vi "UpdateMatlabParamDataToVartiant.vi"(6 "Ignore parent name":bool, 8 "MatlabDataBundle":T1, 9 "curNameIndex":i32, 10 "NamePath":string[](array[string]), 11 "Type (or value to update)":variant) -> (3 "Value":variant)   [LabVIEW 2017]
uses:
  Types/MatlabDataBundle.ctl
  Types/MatlabDataType.ctl
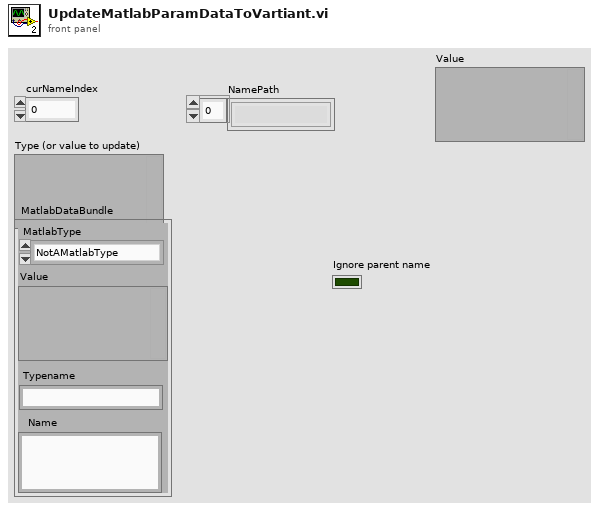
[diagram p1: front panel]
types:
  T1 = typedef "MatlabDataBundle.ctl" = cluster{"MatlabType":T2, "Value":variant, "Name":string, "Typename":string}
  T2 = typedef "MatlabDataType.ctl" = enum16{"NotAMatlabType", "Real", "Complex", "String", "Boolean"}
  T3 = typedef "NI_Data Type.lvlib/Data Type.ctl" = enum8{"Invalid Type", "Void", "I8", "I16", "I32", "I64", "U8", "U16", "U32", "U64", "Single Float", "Double Float", "Extended Float", "Single Complex", "Double Complex", "Extended Complex", "Enum U8", "Enum U16", "Enum U32", "Enum U64", "Single Float With Unit", "Double Float With Unit", "Extended Float With Unit", "Single Complex with Unit", "Double Complex with Unit", "Extended Complex with Unit", "Boolean", "String", "Path", "Picture", "Tag", "Array", "Cluster", "Variant", "LV Variant", "Waveform", "Timestamp", "Digital Waveform", "Digital Data", "ExpressData", "Refnum", "External Data", "VI", "Poly VI", "LabVIEW Class Instance", "Fixed Point"}
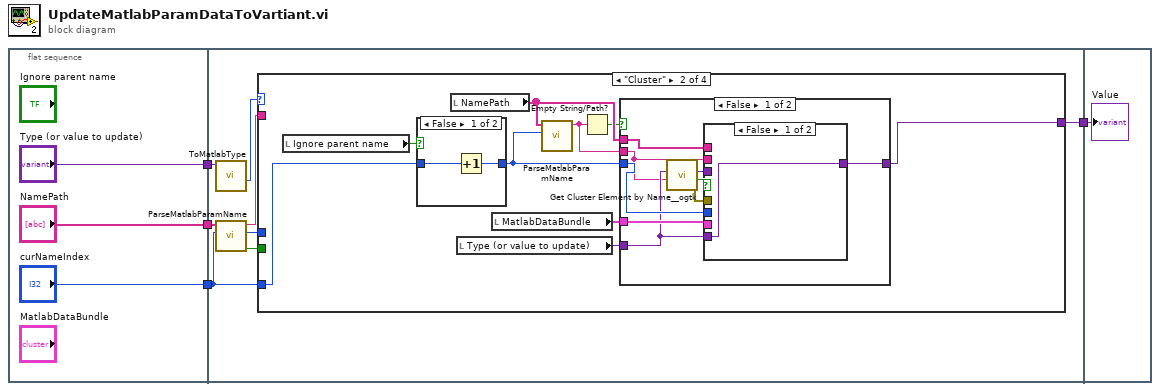
[diagram p0: block diagram]
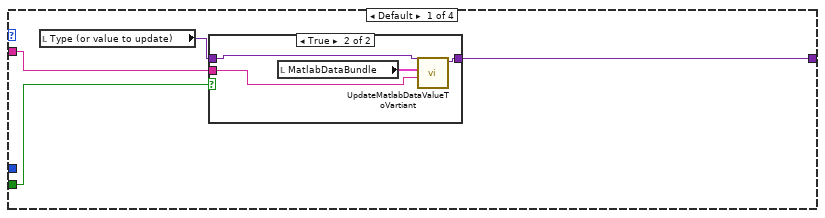
[diagram p2: hidden frame]
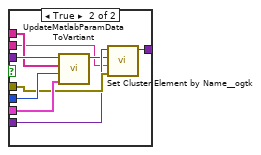
[diagram p4: hidden frame]
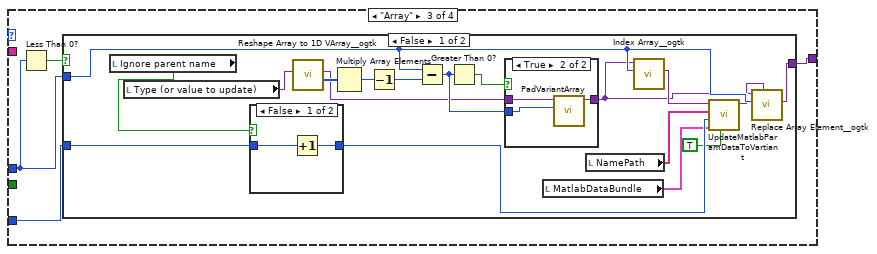
[diagram p7: hidden frame]
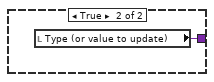
[diagram p10: hidden frame]
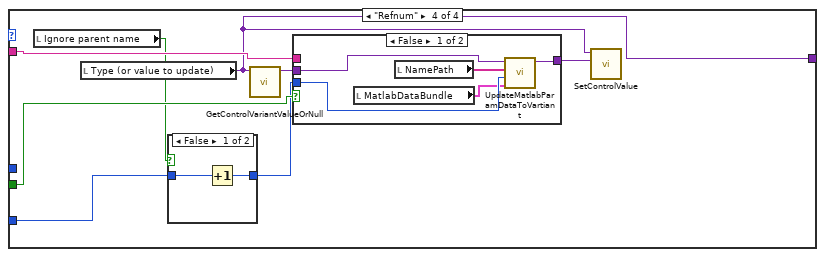
[diagram p11: hidden frame]
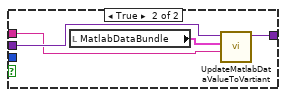
[diagram p13: hidden frame]
diagram:
  n1 = flat-sequence {
    tunnel: ["curNameIndex"] -> w4
    tunnel: ["Type (or value to update)"] -> w3
    tunnel: ["NamePath"] -> w2
    tunnel: w4 -> [w11]
    tunnel: w3 -> [w9]
    tunnel: w2 -> [w10]
    tunnel: [w8] -> w1
    tunnel: w1 -> [w107]
    frame #0 {
    }
    frame #1 {
      n2 = call "ToMatlabType.vi"("Value"=w9) -> ("Type"=w14:T3)  [unwired: 7 in, 3 out]
      n3 = call "ParseMatlabParamName.vi"("curNameIndex"=w11, "NamePath"=w10) -> ("At last name"=w15:bool, "Array Index (or -1)"=w12:i32, "Name"=w13:string)  [unwired: 6 in, 1 out]
      n4 = case shown="\"Cluster\"" w14 {
        tunnel: w15 -> [w18 _ _ w93]
        tunnel: [w19 w27 w59 w87] -> w8
        tunnel: w12 -> [_ _ w58 _]
        tunnel: w13 -> [w17 _ _ w89]
        tunnel: w11 -> [_ w33 w57 w94]
        frame Default {
          n5 = local read "Type (or value to update)"() -> (w16:variant)
          n6 = case shown="True" w18 {
            tunnel: [w20 w24] -> w19
            tunnel: w16 -> [w20 w23]
            tunnel: w17 -> [_ w22]
            frame False {
            }
            frame True {
              n7 = local read "MatlabDataBundle"() -> (w21:T1)
              n8 = call "UpdateMatlabDataValueToVartiant.vi"("name"=w22, "MatlabDataBundle"=w21, "Type (or value to update)"=w23) -> ("Value"=w24:variant)  [unwired: 8 in]
            }
          }
        }
        frame "Cluster" {
          n9 = local read "Ignore parent name"() -> (w30:bool)
          n10 = case shown="False" w30 {
            tunnel: w33 -> [w55 w56]
            tunnel: [w54 w56] -> w32
            frame False {
              n11 = Increment(x=w55) -> (x+1=w54:i32)
            }
            frame True {
            }
          }
          n12 = local read "NamePath"() -> (w29:string[])
          n13 = local read "Type (or value to update)"() -> (w28:variant)
          n14 = local read "MatlabDataBundle"() -> (w31:T1)
          n15 = call "ParseMatlabParamName.vi"("curNameIndex"=w32, "NamePath"=w29) -> ("Name"=w26:string)  [unwired: 6 in, 3 out]
          n16 = Empty String/Path?(string/path=w26) -> (empty?=w25:bool)
          n17 = case shown="False" w25 {
            tunnel: w32 -> [w41 _]
            tunnel: w31 -> [w40 _]
            tunnel: w29 -> [w39 _]
            tunnel: w28 -> [w37 w53]
            tunnel: [w36 w53] -> w27
            tunnel: w26 -> [w35 _]
            frame False {
              n18 = call <userlib>:"Get Cluster Element by Name__ogtk.vi"("Element Name"=w35, "Cluster"=w37) -> ("error out"=w38:errorcluster, "found?"=w34:bool, "VElement"=w42:variant)  [unwired: 7 in]
              n19 = case shown="False" w34 {
                tunnel: w42 -> [_ w52]
                tunnel: w41 -> [_ w51]
                tunnel: w40 -> [_ w50]
                tunnel: w39 -> [_ w49]
                tunnel: w38 -> [_ w48]
                tunnel: w37 -> [w43 w47]
                tunnel: [w43 w46] -> w36
                tunnel: w35 -> [_ w44]
                frame False {
                }
                frame True {
                  n20 = call "UpdateMatlabParamDataToVartiant.vi"("MatlabDataBundle"=w50, "curNameIndex"=w51, "NamePath"=w49, "Type (or value to update)"=w52) -> ("Value"=w45:variant)  [unwired: 7 in]
                  n21 = call <userlib>:"Set Cluster Element by Name__ogtk.vi"("error in (no error)"=w48, "Element Name (\"\": New Element Data Name)"=w44, "New Element Value"=w45, "Cluster"=w47) -> ("VCluster out"=w46:variant)  [unwired: 5 in, 2 out]
                }
              }
            }
            frame True {
            }
          }
        }
        frame "Array" {
          n22 = Less Than 0?(x=w58) -> (x < 0?=w60:bool)
          n23 = case shown="False" w60 {
            tunnel: [w66 w86] -> w59
            tunnel: w58 -> [w72 _]
            tunnel: w57 -> [w70 _]
            frame False {
              n24 = local read "Ignore parent name"() -> (w63:bool)
              n25 = local read "Type (or value to update)"() -> (w61:variant)
              n26 = case shown="False" w63 {
                tunnel: w70 -> [w80 w81]
                tunnel: [w79 w81] -> w69
                frame False {
                  n27 = Increment(x=w80) -> (x+1=w79:i32)
                }
                frame True {
                }
              }
              n28 = call <userlib>:"Reshape Array to 1D VArray__ogtk.vi"("MultiD Array"=w61) -> ("Size(s)"=w74:u32[], "1D VArray"=w73:variant)  [unwired: 8 in, 1 out]
              n29 = Multiply Array Elements(1:w74) -> (0:w78:u32)
              n30 = Decrement(x=w78) -> (x-1=w77:u32)
              n31 = Subtract(x=w72, y=w77) -> (x-y=w75:u32)
              n32 = Greater Than 0?(x=w75) -> (x > 0?=w76:bool)
              n33 = case shown="True" w76 {
                tunnel: w75 -> [_ w85]
                tunnel: w73 -> [w82 w84]
                tunnel: [w82 w83] -> w67
                frame False {
                }
                frame True {
                  n34 = call "PadVariantArray.vi"("PadBy"=w85, "Array In"=w84) -> ("Array out"=w83:variant)  [unwired: 8 in, 1 out]
                }
              }
              n35 = local read "MatlabDataBundle"() -> (w64:T1)
              n36 = local read "NamePath"() -> (w62:string[])
              n37 = call <userlib>:"Index Array__ogtk.vi"("Index (1D)"=w72, "MultiD Array"=w67) -> ("Array Element"=w71:variant)  [unwired: 8 in, 1 out]
              n38 = call "UpdateMatlabParamDataToVartiant.vi"("Ignore parent name"=TRUE, "MatlabDataBundle"=w64, "curNameIndex"=w69, "NamePath"=w62, "Type (or value to update)"=w71) -> ("Value"=w68:variant)  [unwired: 6 in]
              n39 = call <userlib>:"Replace Array Element__ogtk.vi"("New Element"=w68, "Index (1D)"=w72, "MultiD Array"=w67) -> ("VMultiD Array"=w66:variant)  [unwired: 7 in, 1 out]
            }
            frame True {
              n40 = local read "Type (or value to update)"() -> (w86:variant)
            }
          }
        }
        frame "Refnum" {
          n41 = local read "Ignore parent name"() -> (w88:bool)
          n42 = local read "Type (or value to update)"() -> (w87:variant)
          n43 = case shown="False" w88 {
            tunnel: w94 -> [w96 w97]
            tunnel: [w95 w97] -> w92
            frame False {
              n44 = Increment(x=w96) -> (x+1=w95:i32)
            }
            frame True {
            }
          }
          n45 = call "GetControlVariantValueOrNull.vi"("ControlVariant"=w87) -> ("Value"=w91:variant)  [unwired: 9 in, 1 out]
          n46 = case shown="False" w93 {
            tunnel: w92 -> [w102 _]
            tunnel: w91 -> [w101 w106]
            tunnel: [w100 w105] -> w90
            tunnel: w89 -> [_ w104]
            frame False {
              n47 = local read "MatlabDataBundle"() -> (w99:T1)
              n48 = local read "NamePath"() -> (w98:string[])
              n49 = call "UpdateMatlabParamDataToVartiant.vi"("MatlabDataBundle"=w99, "curNameIndex"=w102, "NamePath"=w98, "Type (or value to update)"=w101) -> ("Value"=w100:variant)  [unwired: 7 in]
            }
            frame True {
              n50 = local read "MatlabDataBundle"() -> (w103:T1)
              n51 = call "UpdateMatlabDataValueToVartiant.vi"("name"=w104, "MatlabDataBundle"=w103, "Type (or value to update)"=w106) -> ("Value"=w105:variant)  [unwired: 8 in]
            }
          }
          n52 = call "SetControlValue.vi"("Value"=w90, "ControlVariant"=w87) -> ()  [unwired: 9 in, 1 out]
        }
      }
    }
    frame #2 {
      "Value" <- w107
    }
  }
